vi "SMC_AxisRel.vi"(8 "error in (no error)":errorcluster, 9 "WaitUntilReady":bool, 10 "Distance":dbl format="%.6f", 11 "AxisNr":u8) -> (0 "error out":errorcluster)   [LabVIEW 2015]
doc: "AxisNr is only used in VENUS 1. It is ignored in VENUS 2"
uses:
  SMC_SubVIs.llb/SMC_ManagerMode.ctl
  SMC_SubVIs.llb/glb_stop.vi
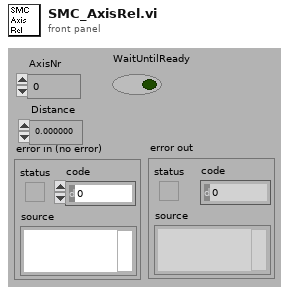
[diagram p1: front panel]
types:
  T1 = typedef "SMC_ManagerMode.ctl" = enum16{"Init", "Get", "SetPosition", "SetStatus", "SetMoving", "SetControllerNr"}
  T2 = typedef "SMC Paras.ctl" = cluster{"VENUS Language":T3, "Number of Axis":u8, "Controller Nr":u8, "Simulation":bool}
  T3 = typedef "VENUSNr.ctl" = enum16{"VENUS 2", "VENUS 1"}
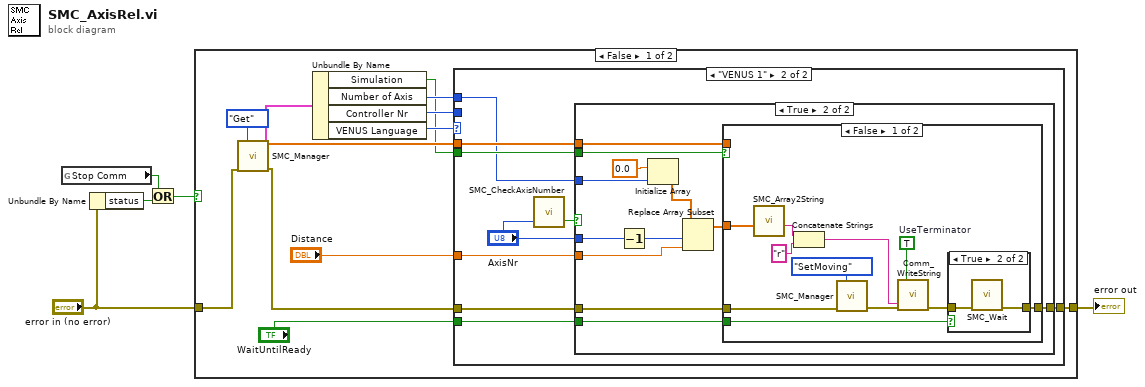
[diagram p0: block diagram]
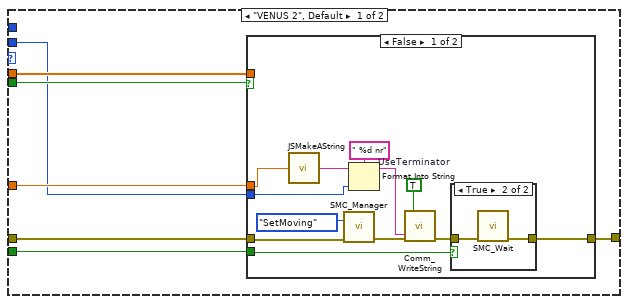
[diagram p2: hidden frame]
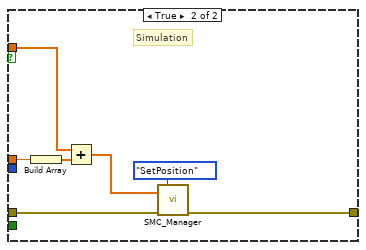
[diagram p4: hidden frame]
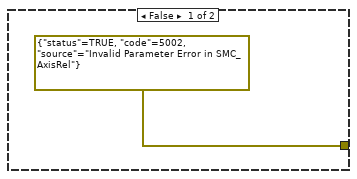
[diagram p5: hidden frame]
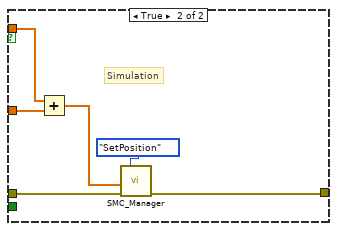
[diagram p7: hidden frame]
diagram:
  n1 = global read "glb_stop.vi" "Stop Comm"() -> (w3:bool)
  n2 = Unbundle By Name("error in (no error)") -> ("status"=w2:bool)
  n3 = Or(x=w3, y=w2) -> (x .or. y?=w1:bool)
  n4 = case shown="False" w1 {
    tunnel: "error in (no error)" -> [w16 w89]
    tunnel: [w15 w89] -> w4
    frame False {
      n5 = call "SMC_Manager.vi"("Mode"=SMC_ManagerMode."Get", "error in (no error)"=w16) -> ("SMC Parameter Out"=w10:T2, "Position"=w13:dbl[], "error out"=w14:errorcluster)  [unwired: 9 in, 2 out]
      n6 = Unbundle By Name(w10) -> ("Simulation"=w6:bool, "Number of Axis"=w7:u8, "Controller Nr"=w8:u8, "VENUS Language"=w9:T3)
      n7 = case shown="\"VENUS 1\"" w9 {
        tunnel: [w22 w55] -> w15
        tunnel: w14 -> [w23 w54]
        tunnel: w6 -> [w24 w53]
        tunnel: w13 -> [w21 w50]
        tunnel: "Distance" -> [w20 w49]
        tunnel: "WaitUntilReady" -> [w19 w48]
        tunnel: w8 -> [w18 _]
        tunnel: w7 -> [_ w47]
        frame "VENUS 2", Default {
          n8 = case shown="False" w24 {
            tunnel: w23 -> [w35 w45]
            tunnel: [w28 w44] -> w22
            tunnel: w21 -> [_ w43]
            tunnel: w20 -> [w27 w41]
            tunnel: w18 -> [w32 _]
            tunnel: w19 -> [w30 _]
            frame False {
              w25 = TRUE  # UseTerminator
              n9 = call "JSMakeAString.vi"("Value"=w27) -> ("String"=w26:string)
              n10 = call "SMC_Manager.vi"("Mode"=SMC_ManagerMode."SetMoving", "error in (no error)"=w35) -> ("error out"=w36:errorcluster)  [unwired: 9 in, 4 out]
              n11 = Format Into String(format string=" %d nr" ("Format String"), initial string=w26, w32) -> (resulting string=w31:string)  [unwired: 1 in, 1 out]
              n12 = call "Comm_WriteString.vi"("string to write"=w31, "error in (no error)"=w36, "UseTerminator"=w25) -> ("error out"=w29:errorcluster)  [unwired: 8 in]
              n13 = case shown="True" w30 {
                tunnel: w29 -> [w37 w39]
                tunnel: [w37 w38] -> w28
                frame False {
                }
                frame True {
                  n14 = call "SMC_Wait.vi"("error in (no error)"=w39) -> ("error out"=w38:errorcluster)  [unwired: 10 in]
                }
              }
            }
            frame True {
              # "Simulation"
              n15 = Build Array(w41) -> (w42:dbl[])
              n16 = Add(x=w43, y=w42) -> (x+y=w40:dbl[])
              n17 = call "SMC_Manager.vi"("Mode"=SMC_ManagerMode."SetPosition", "PosArraySimu"=w40, "error in (no error)"=w45) -> ("error out"=w44:errorcluster)  [unwired: 8 in, 4 out]
            }
          }
        }
        frame "VENUS 1" {
          n18 = call "SMC_CheckAxisNumber.vi"("AxisNr"="AxisNr") -> ("Result"=w51:bool)  [unwired: 10 in]
          n19 = case shown="True" w51 {
            tunnel: "AxisNr" -> [_ w66]
            tunnel: w47 -> [_ w65]
            tunnel: w54 -> [_ w63]
            tunnel: [errorcluster {"status"=TRUE, "code"=5002, "source"="Invalid Parameter Error in SMC_AxisRel"} ("t") w64] -> w55
            tunnel: w53 -> [_ w62]
            tunnel: w50 -> [_ w61]
            tunnel: w49 -> [_ w60]
            tunnel: w48 -> [_ w57]
            frame False {
            }
            frame True {
              n20 = Decrement(x=w66) -> (x-1=w68:u8)
              n21 = Initialize Array(0.0 ("Element Data"), w65) -> (w58:dbl[])
              n22 = Replace Array Subset(array=w58, new element=w60, index=w68) -> (w67:dbl[])
              n23 = case shown="False" w62 {
                tunnel: w67 -> [w74 w87]
                tunnel: [w71 w84] -> w64
                tunnel: w63 -> [w75 w85]
                tunnel: w61 -> [_ w88]
                tunnel: w57 -> [w70 _]
                frame False {
                  w69 = TRUE  # UseTerminator
                  n24 = call "SMC_Array2String.vi"("Input Array"=w74) -> ("String"=w73:string)  [unwired: 10 in]
                  n25 = Concatenate Strings(w73, "r" ("Substring")) -> (w78:string)
                  n26 = call "SMC_Manager.vi"("Mode"=SMC_ManagerMode."SetMoving", "error in (no error)"=w75) -> ("error out"=w76:errorcluster)  [unwired: 9 in, 4 out]
                  n27 = call "Comm_WriteString.vi"("string to write"=w78, "error in (no error)"=w76, "UseTerminator"=w69) -> ("error out"=w72:errorcluster)  [unwired: 8 in]
                  n28 = case shown="True" w70 {
                    tunnel: w72 -> [w80 w82]
                    tunnel: [w80 w81] -> w71
                    frame False {
                    }
                    frame True {
                      n29 = call "SMC_Wait.vi"("error in (no error)"=w82) -> ("error out"=w81:errorcluster)  [unwired: 10 in]
                    }
                  }
                }
                frame True {
                  # "Simulation"
                  n30 = Add(x=w88, y=w87) -> (x+y=w83:dbl[])
                  n31 = call "SMC_Manager.vi"("Mode"=SMC_ManagerMode."SetPosition", "PosArraySimu"=w83, "error in (no error)"=w85) -> ("error out"=w84:errorcluster)  [unwired: 8 in, 4 out]
                }
              }
            }
          }
        }
      }
    }
    frame True {
      # "Error, do nothing"
    }
  }
  "error out" <- w4
